vi "Sequence2.vi"(6 "speed":dbl=0.7, 8 "AI 7 Feedback (inches)":dbl, 9 "AI 7 PWM Input":dbl, 10 "AI 5 Setpoint Secondary":dbl, 11 "AI 5 PWM Input":dbl) -> (2 "AI 7 PWM Output":dbl, 3 "AI 5 PWM Output":dbl)   [LabVIEW 2011]
uses:
  Robot Global Data.vi
panel:
  out "AI 7 Previous":dbl
  in  "Forced Retraction":dbl
  in  "Rotation Sequence":dbl
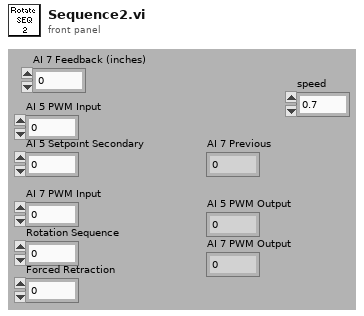
[diagram p1: front panel]
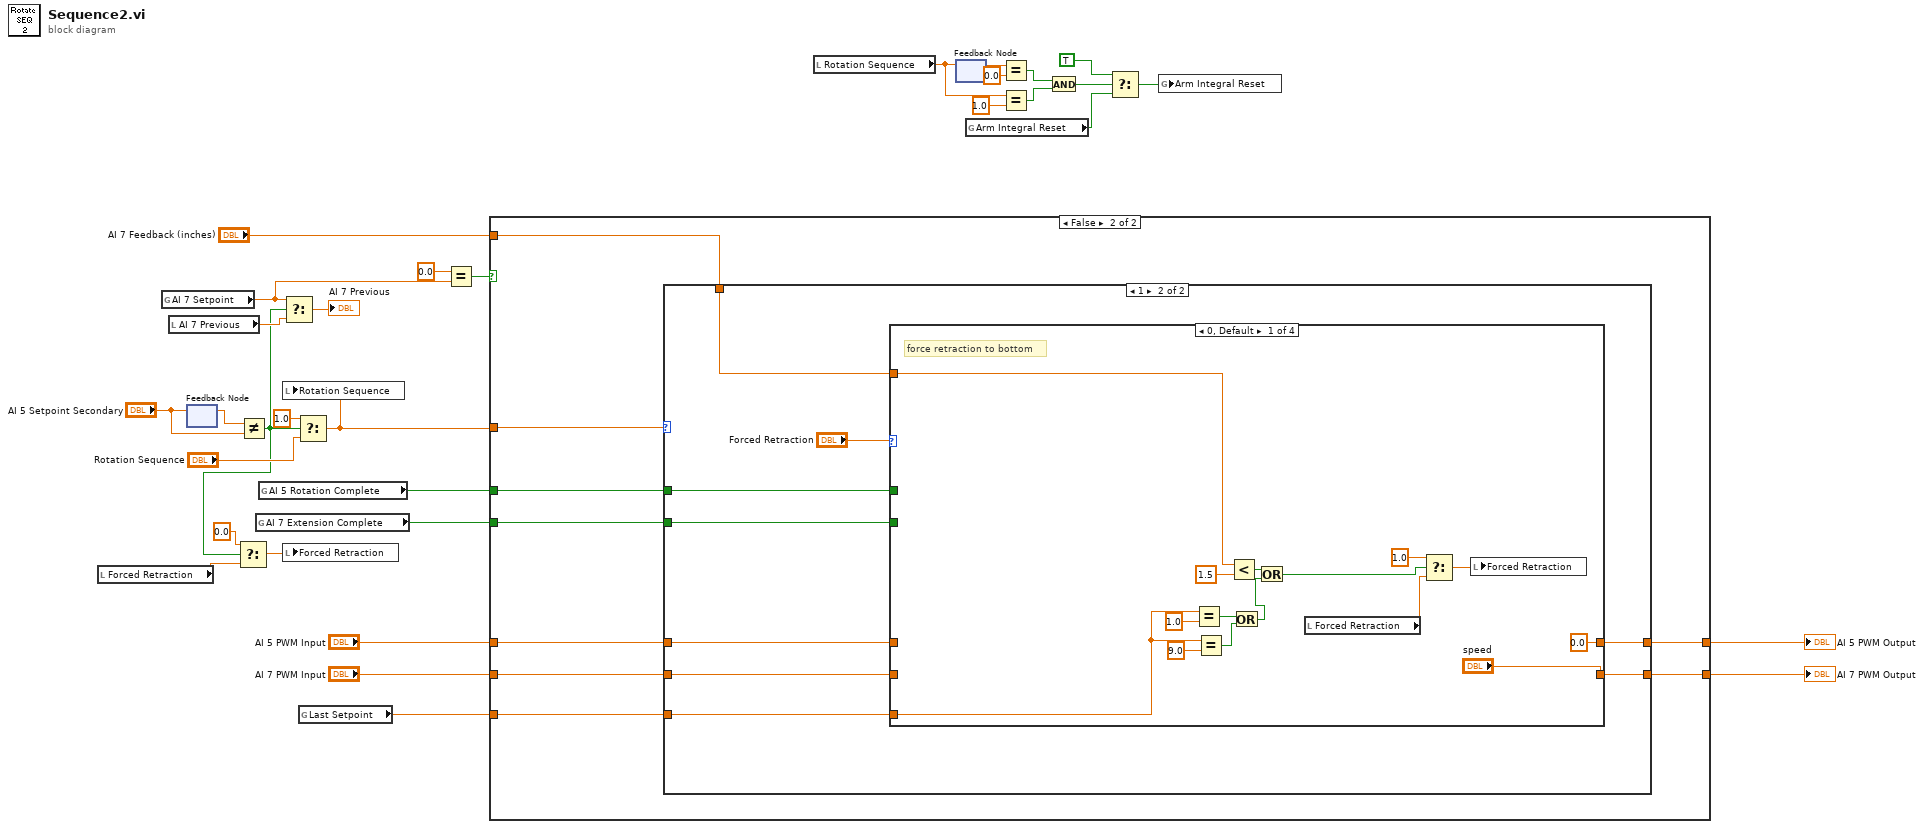
[diagram p0: block diagram]
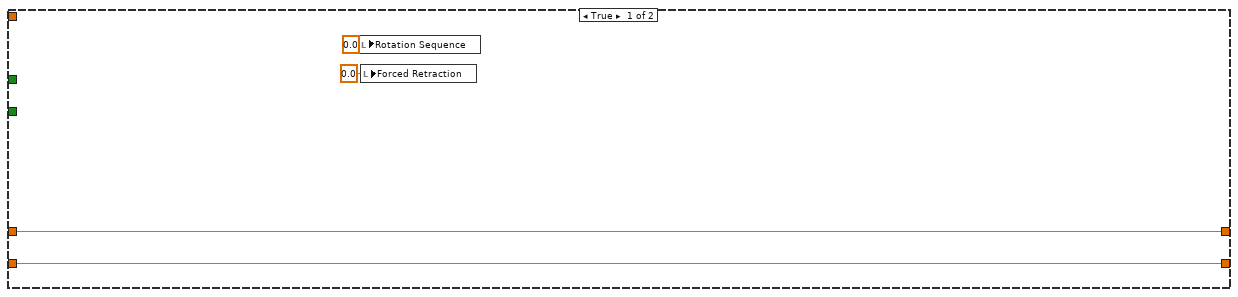
[diagram p2: hidden frame]
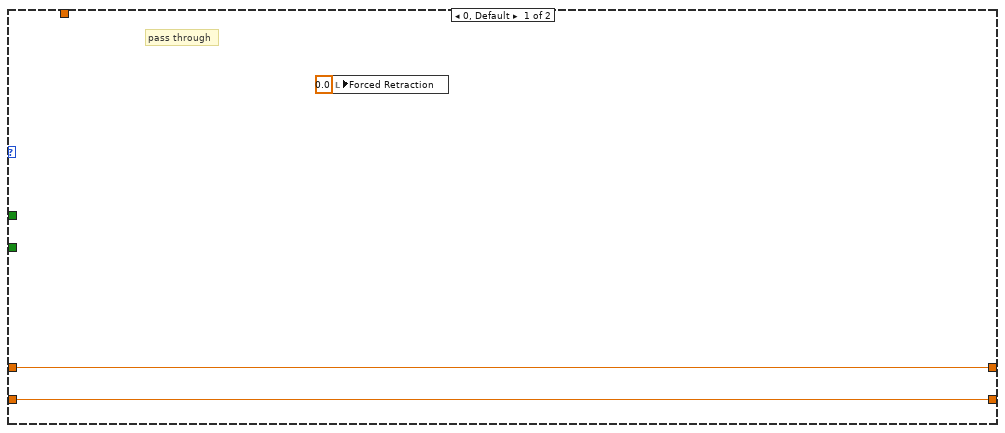
[diagram p3: hidden frame]
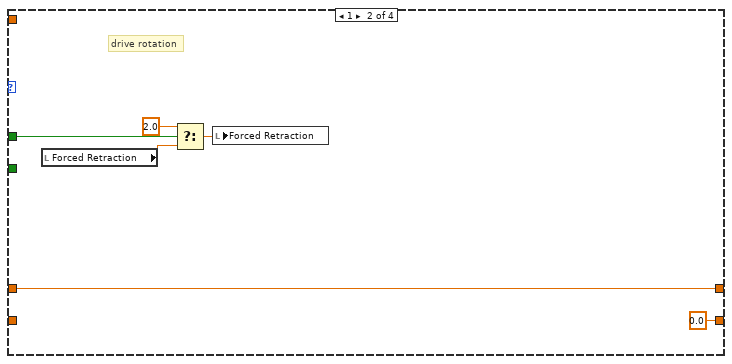
[diagram p4: hidden frame]
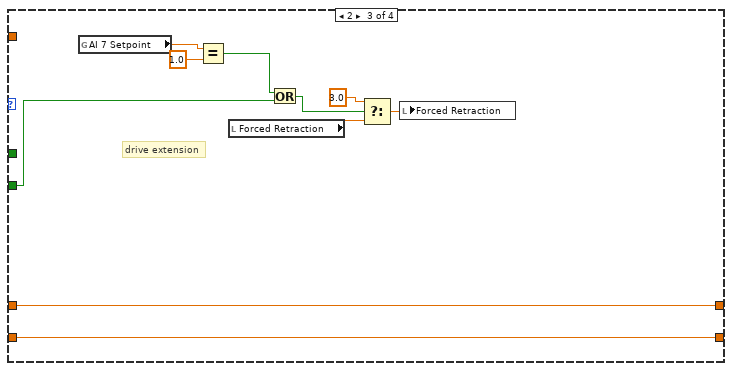
[diagram p5: hidden frame]
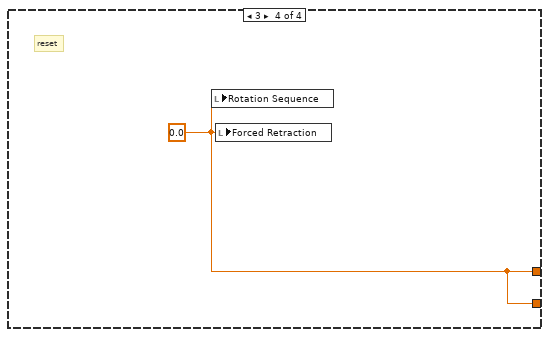
[diagram p6: hidden frame]
diagram:
  n1 = local read "Forced Retraction"() -> (w6:dbl)
  n2 = global read "Robot Global Data.vi" "AI 7 Setpoint"() -> (w2:dbl)
  n3 = local read "AI 7 Previous"() -> (w22:dbl)
  n4 = feedback-in #1("AI 5 Setpoint Secondary") -> ()
  n5 = feedback #1() -> (w32:dbl)  [unwired: 1 out]
  n6 = Not Equal?(x=w32, y="AI 5 Setpoint Secondary") -> (x != y?=w8:bool)
  n7 = Select(t=0.0, s=w8, f=w6) -> (s? t:f=w5:dbl)
  n8 = global read "Robot Global Data.vi" "AI 7 Extension Complete"() -> (w10:bool)
  n9 = global read "Robot Global Data.vi" "AI 5 Rotation Complete"() -> (w21:bool)
  n10 = local write "Forced Retraction"(w5) -> ()
  n11 = Select(t=w2, s=w8, f=w22) -> (s? t:f=→"AI 7 Previous":dbl)
  n12 = Select(t=1.0, s=w8, f="Rotation Sequence") -> (s? t:f=w24:dbl)
  n13 = local write "Rotation Sequence"(w24) -> ()
  n14 = global read "Robot Global Data.vi" "Last Setpoint"() -> (w4:dbl)
  n15 = Equal?(x=0.0, y=w2) -> (x = y?=w3:bool)
  n16 = case shown="False" w3 {
    tunnel: "AI 5 PWM Input" -> [w36 w45]
    tunnel: "AI 7 PWM Input" -> [w35 w44]
    tunnel: [w36 w43] -> w27
    tunnel: [w35 w42] -> w26
    tunnel: w24 -> [_ w41]
    tunnel: w21 -> [_ w40]
    tunnel: w10 -> [_ w39]
    tunnel: "AI 7 Feedback (inches)" -> [_ w38]
    tunnel: w4 -> [_ w37]
    frame True {
      n17 = local write "Rotation Sequence"(0.0 ("Rotation Sequence")) -> ()
      n18 = local write "Forced Retraction"(0.0 ("Forced Retraction")) -> ()
    }
    frame False {
      n19 = case shown="1" w41 {
        tunnel: w45 -> [w48 w53]
        tunnel: w44 -> [w47 w57]
        tunnel: [w48 w54] -> w43
        tunnel: [w47 w56] -> w42
        tunnel: w40 -> [_ w52]
        tunnel: w39 -> [_ w51]
        tunnel: w38 -> [_ w50]
        tunnel: w37 -> [_ w49]
        frame 0, Default {
          # "pass through"
          n20 = local write "Forced Retraction"(0.0 ("Forced Retraction")) -> ()
        }
        frame 1 {
          n21 = case shown="0, Default" "Forced Retraction" {
            tunnel: w57 -> [_ _ w87 _]
            tunnel: ["speed" 0.0 ("AI 7 PWM Input") w87 w89] -> w56
            tunnel: [0.0 ("AI 5 PWM Input") w77 w88 w89] -> w54
            tunnel: w53 -> [_ w77 w88 _]
            tunnel: w52 -> [_ w76 _ _]
            tunnel: w51 -> [_ _ w82 _]
            tunnel: w50 -> [w70 _ _ _]
            tunnel: w49 -> [w59 _ _ _]
            frame 0, Default {
              # "force retraction to bottom"
              n22 = Equal?(x=w59, y=1.0) -> (x = y?=w62:bool)
              n23 = Equal?(x=w59, y=9.0) -> (x = y?=w61:bool)
              n24 = Less?(x=w70, y=1.5) -> (x < y?=w66:bool)
              n25 = Or(x=w62, y=w61) -> (x .or. y?=w60:bool)
              n26 = Or(x=w66, y=w60) -> (x .or. y?=w63:bool)
              n27 = local read "Forced Retraction"() -> (w68:dbl)
              n28 = Select(t=1.0, s=w63, f=w68) -> (s? t:f=w69:dbl)
              n29 = local write "Forced Retraction"(w69) -> ()
            }
            frame 1 {
              # "drive rotation"
              n30 = local read "Forced Retraction"() -> (w74:dbl)
              n31 = Select(t=2.0, s=w76, f=w74) -> (s? t:f=w73:dbl)
              n32 = local write "Forced Retraction"(w73) -> ()
            }
            frame 2 {
              # "drive extension"
              n33 = global read "Robot Global Data.vi" "AI 7 Setpoint"() -> (w81:dbl)
              n34 = Equal?(x=w81, y=1.0 ("t")) -> (x = y?=w80:bool)
              n35 = local read "Forced Retraction"() -> (w85:dbl)
              n36 = Or(x=w80, y=w82) -> (x .or. y?=w83:bool)
              n37 = Select(t=3.0, s=w83, f=w85) -> (s? t:f=w84:dbl)
              n38 = local write "Forced Retraction"(w84) -> ()
            }
            frame 3 {
              w89 = 0.0 ("Forced Retraction")
              # "reset"
              n39 = local write "Rotation Sequence"(w89) -> ()
              n40 = local write "Forced Retraction"(w89) -> ()
            }
          }
        }
      }
    }
  }
  "AI 5 PWM Output" <- w27
  "AI 7 PWM Output" <- w26
  n41 = local read "Rotation Sequence"() -> (w18:dbl)
  n42 = feedback-in #2(w18) -> ()
  n43 = feedback #2() -> (w20:dbl)  [unwired: 1 out]
  n44 = global read "Robot Global Data.vi" "Arm Integral Reset"() -> (w12:bool)
  n45 = Equal?(x=w20, y=0.0) -> (x = y?=w15:bool)
  n46 = Equal?(x=w18, y=1.0) -> (x = y?=w16:bool)
  n47 = And(x=w15, y=w16) -> (x .and. y?=w14:bool)
  n48 = Select(t=TRUE, s=w14, f=w12) -> (s? t:f=w11:bool)
  n49 = global write "Robot Global Data.vi" "Arm Integral Reset"(w11) -> ()
